vi "pirometer 2.2_MAIN.vi"() -> ()   [LabVIEW 2013]
doc: "Пирометр 2.0, разработан в ЛФВЭ ОИЯИ 2013"
uses:
  pirometer typedef1.ctl
  <vilib>/Utility/error.llb/DialogType.ctl
  <vilib>/Instr/_visa.llb/VISA Configure Serial Port (Instr).vi
  <vilib>/ptbypt/NI_PtbyPt.lvlib
panel:
  in  "Бод.":u32=9600
  out "Ошибка  прибора":bool
  in  "Недопустимая \nразница между\n показаниями":u8=100
  in  "Снимок экрана":bool
  in  "Мин\n  d/dt":dbl=-0.02 min=-200.0 max=200.0 step=0.01 format="%#.3g"
  in  "Макс\n  d/dt":dbl=0.02 min=-200.0 max=200.0 step=0.01 format="%#.3g"
  out "d/dt right scale":dbl(slide) min=-0.20900000000000002 max=0.196 scale=-0.02..0.02
  out "gradusnik 2":dbl(slide) scale=10.0..35.0
  in  "Мин. Т":i8=10
  in  "Stop":bool
  out "gradusnik":dbl(slide) scale=10.0..35.0
  in  "Усреднение d/dt":u16=25
  in  "Усреднение T по":u8=50
  out "Средняя T":dbl format="%0.2f"
  out "d/dt":dynamicdata(graph)
  in  "Макс.Т":i8=35
  out "Температура":dynamicdata(graph)
  in  "Запись в файл":bool
  out "сек.":string="20"
  out "мин.":string="3"
  out "часы":string
  in  "xScale +":bool
  in  "Добавить время":dbl(ring)=60.0 items=["1 сек."=1.0, "10 сек."=10.0, "1 мин."=60.0, "5 мин."=300.0, "10 мин."=600.0]
  in  "xScale -":bool
  out "Текущая T":dbl format="%0.2f"
  in  "Порт":refnum<visa-resource-name>="COM4"
  out "Соединение":bool
  out "Чтение":bool
  out "Расположение файла":path=path "Запись в файл не включена..."
  out "d/dt":dbl format="%#.3f"
  in  "2 или 1 ?":bool=TRUE
  out "Exitting":string="Остановка программы..."
  in  "index of current arr element":i32
  out "i":i32
  in  "number of data sample":u64
  out "refnum out":refnum<file>
  in  "fl_1":bool
  out "Temper.":dbl
  out "Err msg":string=" INSTRUCTIONS:\r\rNormal Use:  When using subVIs that incorporate the error in/error out (or error I/O) structure, place this handler where you want to inform the user of an error, typically at the end of the I/O data path, as the last action of the program.  If the error in error? is ERROR, the handler creates a message describing the error and its source.  If the type of dialog = 1 (default), the message is displayed to the user, who can only acknowedge it.  If the type = 2, the user can acknowledge the message or abort execution; aborting a program with active I/O is not recommended.  If the type = 0, no message is displayed; this is used to process the error programmatically, and the error out cluster elements are wired to individual terminals for that reason.  \r\rOther Use:\n\r\nlocal testing.  To test the error code of a subVI or function that does not have the error I/O structure, you can wire its error code and a source string to the local error code and error source inputs.  If error in error? indicates no error and error code is not equal to 0, the local code and source are substituted for the error in values, and error? is set TRUE (ERROR)."
  # "Показывать два графика?"
  # "°С"
  # "°С"
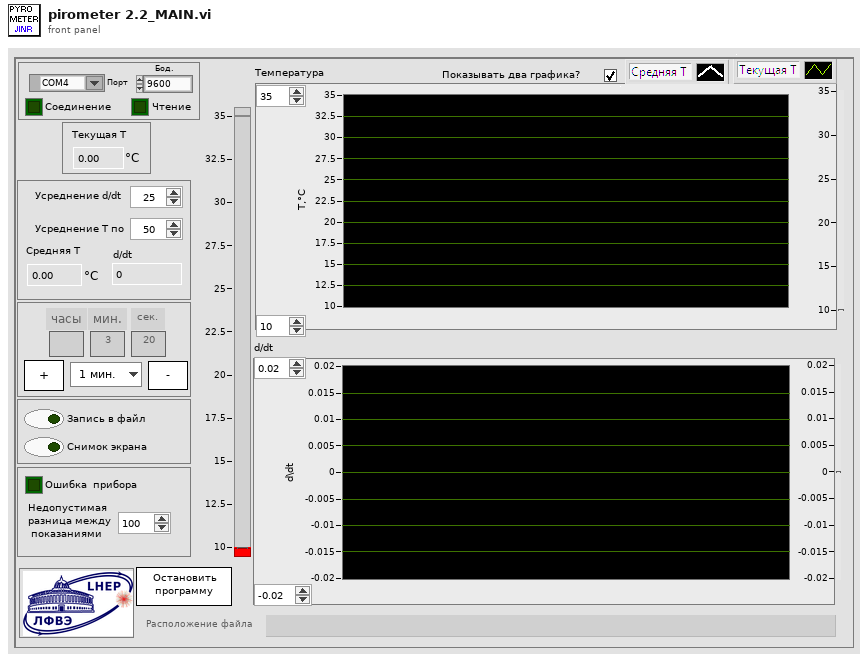
[diagram p1: front panel]
types:
  T1 = typedef "pirometer typedef1.ctl" = enum16{"Initialize", "Read port", "Averaging", "Create graph", "Save to file", "Stop", "ScreenCapture", "Err handle"}
  T2 = typedef "DialogType.ctl" = u16
  T3 = typedef "imagedata.ctl" = cluster{"image type":i32, "image depth":i32, "image":u8[], "mask":u8[], "colors":u32[], "Rectangle":cluster{"left":i16, "top":i16, "right":i16, "bottom":i16}}
  T4 = typedef "LVDateTimeRec.ctl" = cluster{"fractional second":dbl, "second":i32, "minute":i32, "hour":i32, "day of month":i32, "month":i32, "year":i32, "day of week":i32, "day of year":i32, "DST":i32}
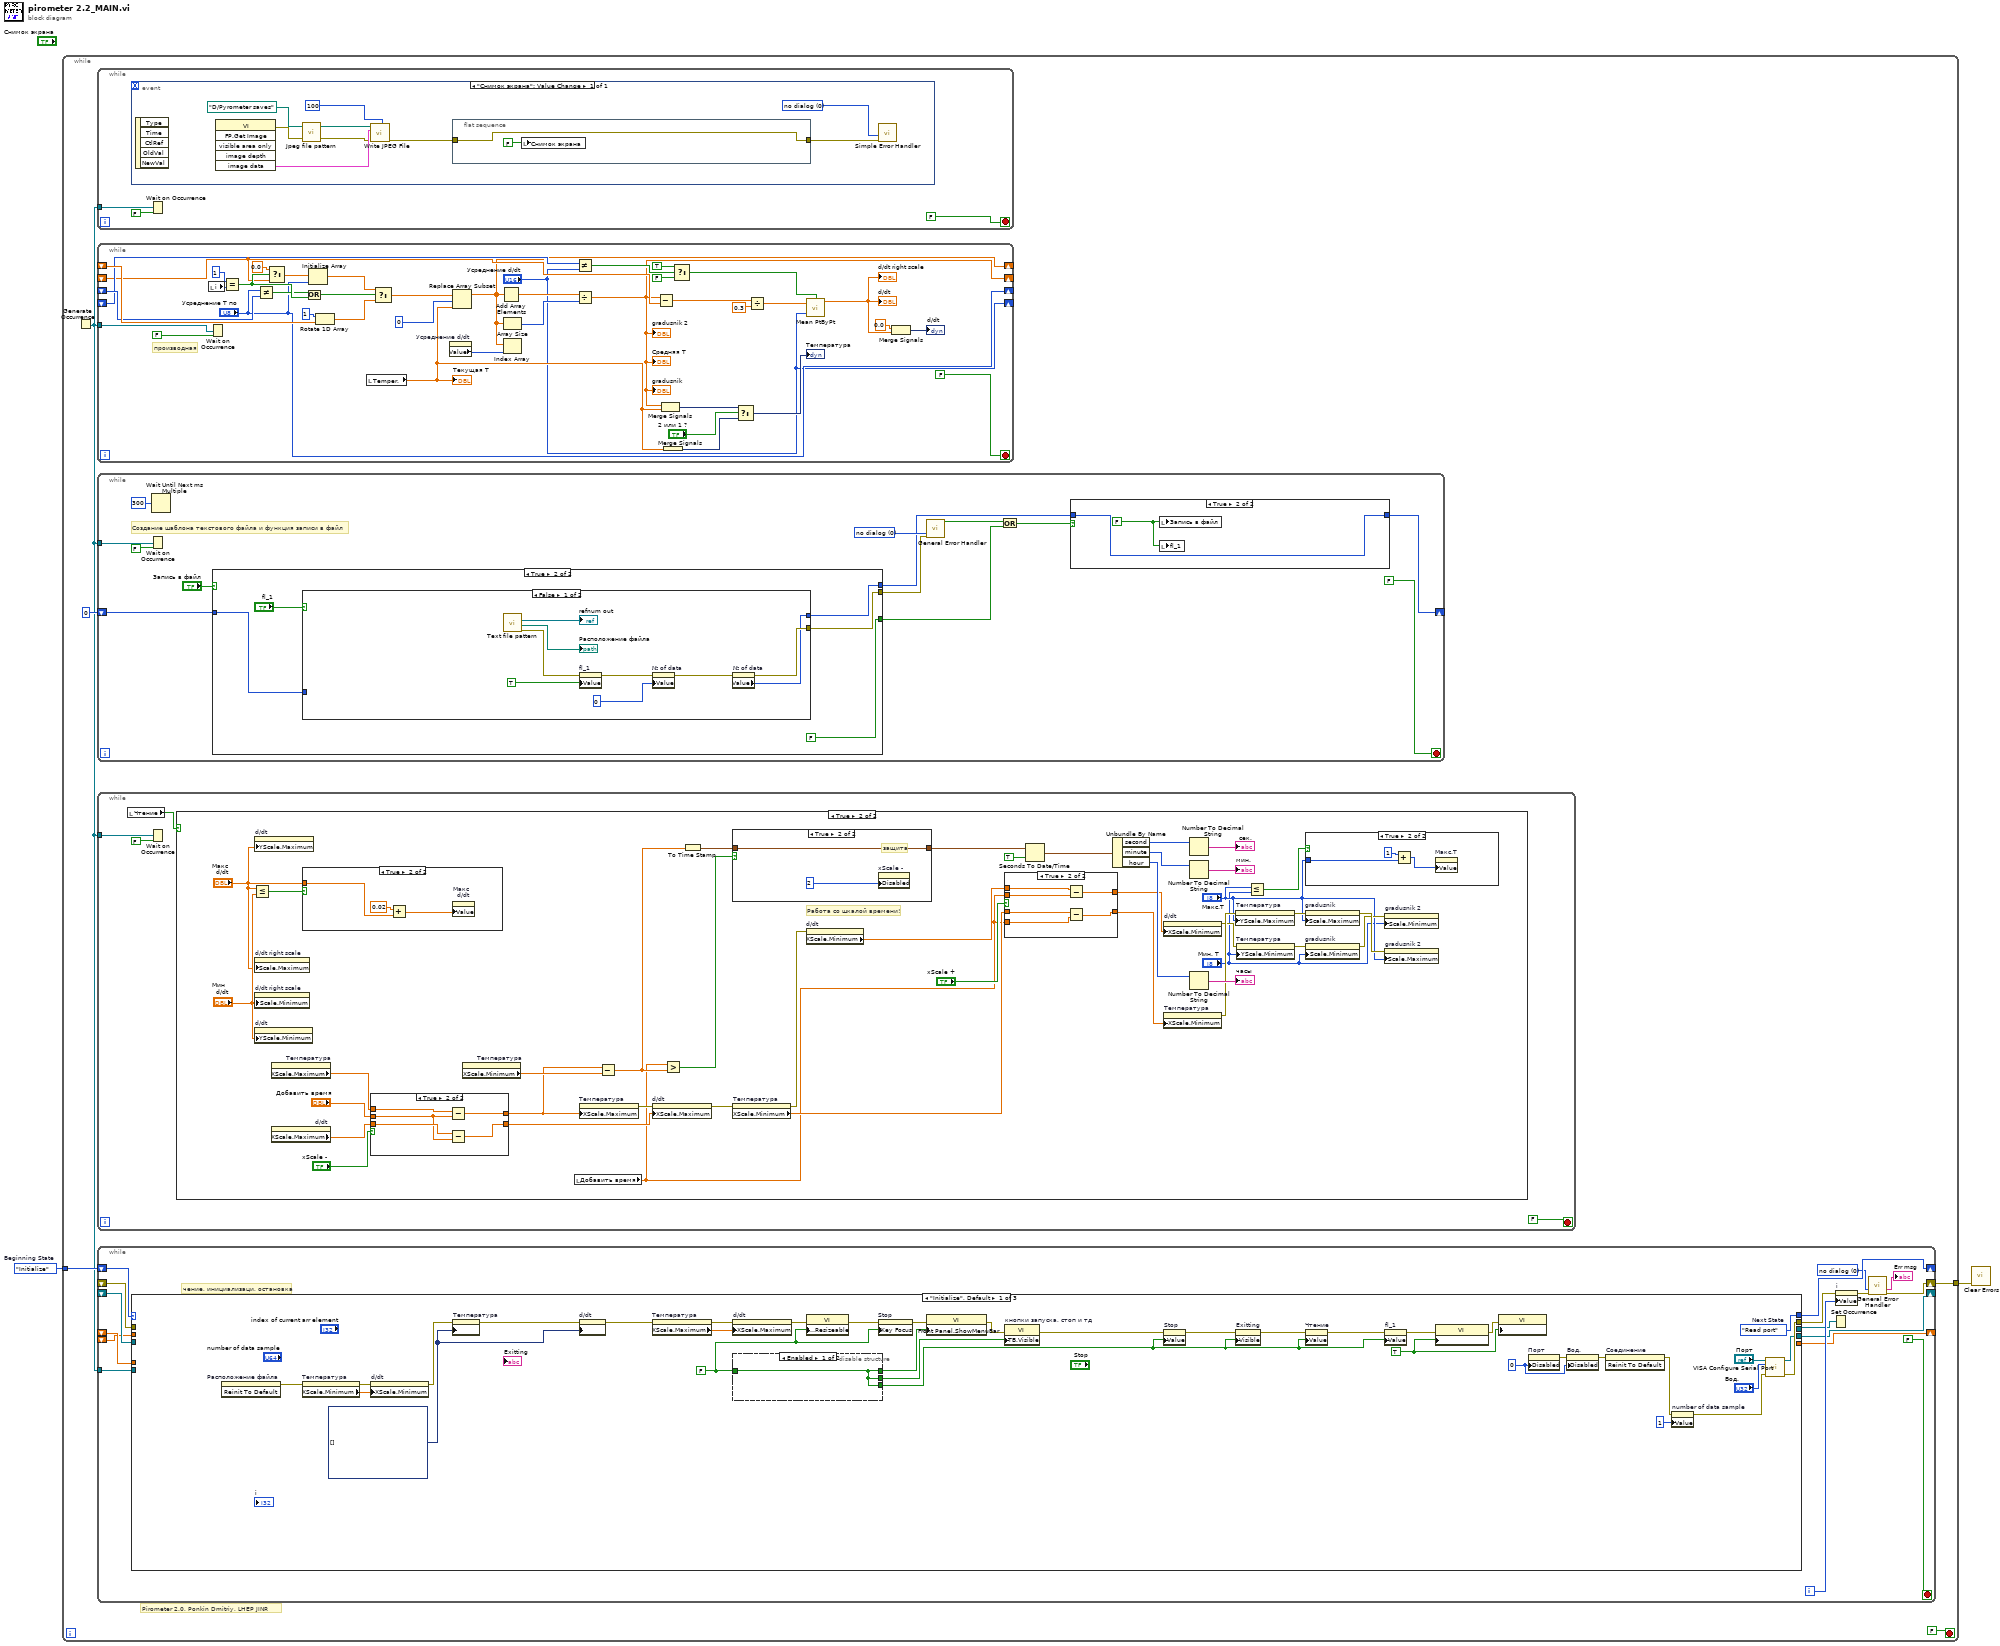
[diagram p0: block diagram]
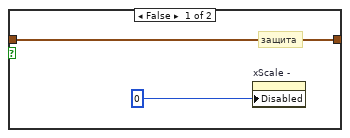
[diagram p5: hidden frame]
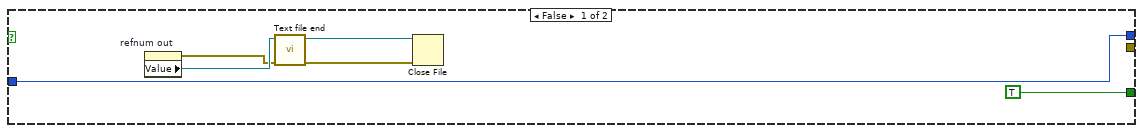
[diagram p9: hidden frame]
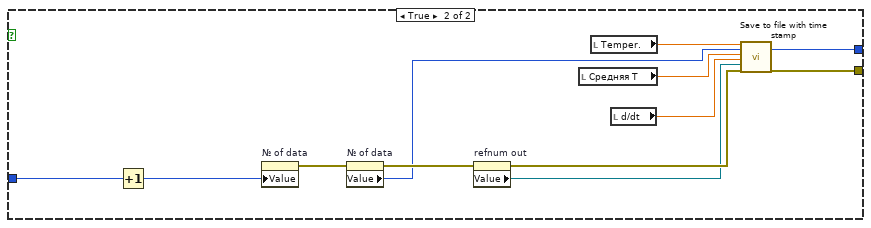
[diagram p10: hidden frame]
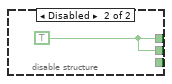
[diagram p11: hidden frame]
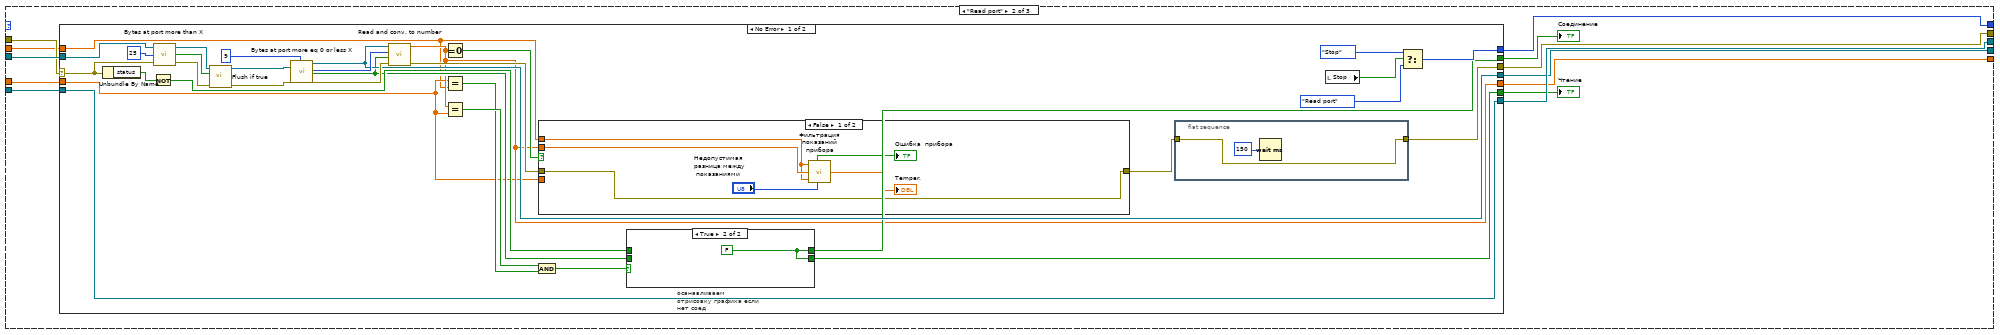
[diagram p12: hidden frame]
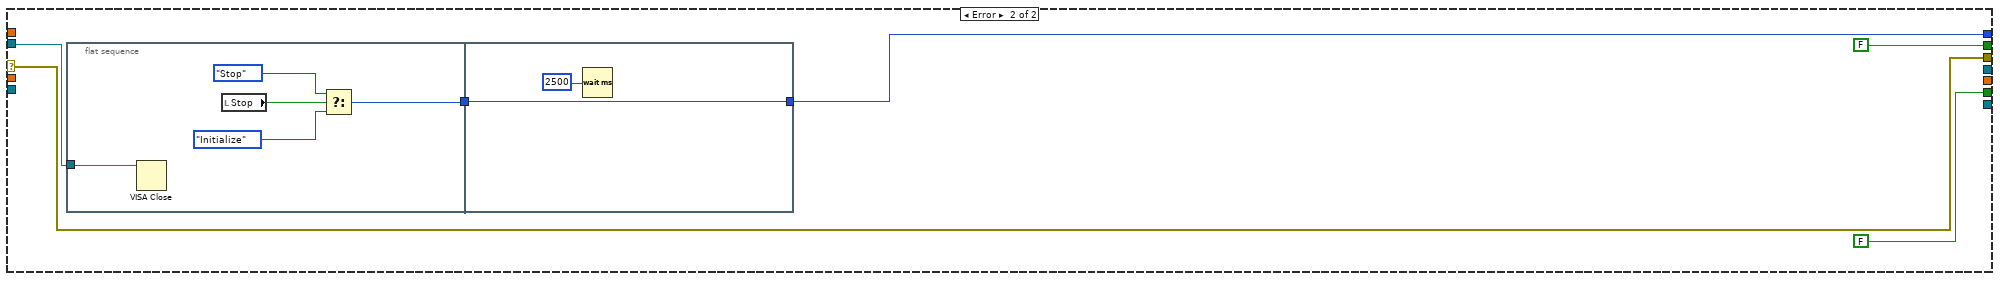
[diagram p15: hidden frame]
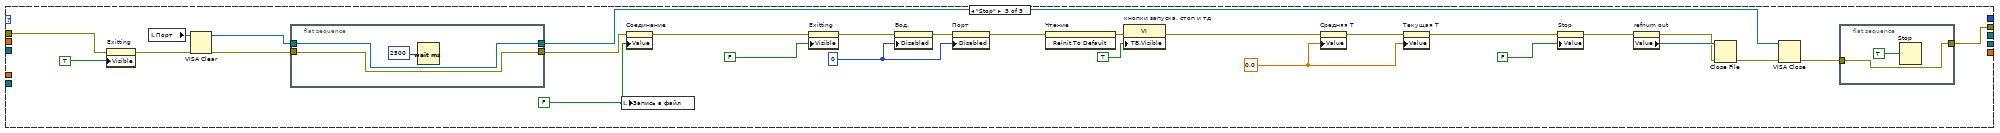
[diagram p16: hidden frame]
diagram:
  w2 = pirometer_typedef1."Initialize"  # Beginning State
  n1 = while {
    tunnel: w2 -> [w7]
    tunnel: [w5] -> w1
    stop <- FALSE stop-if-true
    # "Pirometer 2.0, Ponkin Dmitriy, LHEP JINR"
    n2 = Generate Occurrence() -> (w3:refnum<k4>)
    n3 = while {
      tunnel: w3 -> [w8]
      stop <- FALSE stop-if-true
      n4 = event shown="[0] \"Снимок экрана\": Value Change" {
        selector: _ -> [_]
        dyn-events: _ -> [_]
        timeout: _ -> [_]
        event "Снимок экрана": Value Change {
          w12 = T2 0 items=["no dialog", "OK message", "continue or stop message", "OK message + warnings", "continue/stop + warnings"] ("type of dialog (OK msg:1)")
          n5 = event-data() -> ()  [unwired: 6 out]
          n6 = invoke class="VI" method="FP.Get Image"() -> (error out=w17:errorcluster, "image data"=w18:T3)  [unwired: 6 in, 4 out]
          n7 = call "Jpeg file pattern.vi"("path"=path "D:/Pyrometer saves", "error in"=w17) -> ("path to JPG file"=w16:path, "error out"=w15:errorcluster)  [unwired: 6 out]
          n8 = call <vilib>:"Write JPEG File.vi"("quality (80)"=100, "error in (no error)"=w15, "image data"=w18, "path to JPEG file"=w16) -> ("error out"=w13:errorcluster)  [unwired: 7 out]
          n9 = flat-sequence {
            tunnel: w13 -> [w20]
            tunnel: [w20] -> w11
            frame #0 {
              n10 = local write "Снимок экрана"(FALSE ("Снимок экрана")) -> ()
            }
          }
          n11 = call <vilib>:"Simple Error Handler.vi"("type of dialog (OK msg:1)"=w12, "error in (no error)"=w11) -> ()  [unwired: 8 out]
        }
      }
      n12 = Wait on Occurrence(1:FALSE ("ignore previous (T)"), 2:w8) -> ()  [unwired: 1 in, 1 out]
    }
    n13 = while {
      shift-right: [w24] -> _
      shift-left: _ -> [w62]
      tunnel: w3 -> [w59]
      shift-right: ["Усреднение T по"] -> _
      shift-left: _ -> [w54]
      shift-right: [w30] -> _
      shift-left: _ -> [w31]
      shift-right: ["Усреднение d/dt"] -> _
      shift-left: _ -> [w33]
      stop <- FALSE stop-if-true
      # "производная"
      n14 = local read "i"() -> (w27:i32)
      n15 = Wait on Occurrence(1:FALSE ("ignore previous (T)"), 2:w59) -> ()  [unwired: 1 in, 1 out]
      n16 = Equal?(x=1 ("y"), y=w27) -> (x = y?=w52:bool)
      n17 = Not Equal?(x="Усреднение T по", y=w54) -> (x != y?=w49:bool)
      n18 = Select(t=0.0, s=w52, f=w31) -> (s? t:f=w50:dbl)
      n19 = Or(x=w49, y=w52) -> (x .or. y?=w48:bool)
      n20 = Initialize Array(w50, "Усреднение T по") -> (w43:dbl[])
      n21 = Rotate 1D Array(1:w62, 2:1 ("n")) -> (0:w45:dbl[])
      n22 = local read "Temper."() -> (w40:dbl)
      "Текущая T" <- w40
      n23 = Select(t=w43, s=w48, f=w45) -> (s? t:f=w26:dbl[])
      n24 = property on="Усреднение d/dt" class="DigNum (strict)"() -> ("Value"=w25:u16)  [unwired: 2 in, 2 out]
      n25 = Replace Array Subset(array=w26, new element=w40, index=0) -> (w24:dbl[])
      n26 = Add Array Elements(numeric array=w24) -> (sum=w53:dbl)
      n27 = Array Size(array=w24) -> (size(s)=w29:i32)
      n28 = Index Array(array=w24, index=w25) -> ()  [unwired: 1 out]
      n29 = Not Equal?(x=w33, y="Усреднение d/dt") -> (x != y?=w34:bool)
      n30 = Divide(x=w53, y=w29) -> (x/y=w30:dbl)
      "Средняя T" <- w30
      "gradusnik" <- w30
      "gradusnik 2" <- w30
      n31 = Subtract(x=w30, y=w31) -> (x-y=w42:dbl)
      n32 = Merge Signals(w30, w40) -> (w58:dynamicdata)
      n33 = Merge Signals(w40) -> (w57:dynamicdata)
      n34 = Select(t=TRUE ("initialize"), s=w34, f=FALSE ("initialize")) -> (s? t:f=w32:bool)
      n35 = Select(t=w58, s="2 или 1 ?", f=w57) -> (s? t:f=→"Температура":dynamicdata)
      n36 = Divide(x=w42, y=0.3 ("dT")) -> (x/y=w37:dbl)
      n37 = call <vilib>:"Mean PtByPt.vi"("x"=w37, "sample length"="Усреднение d/dt", "initialize"=w32) -> ("mean"=w38:dbl)  [unwired: 2 out]
      "d/dt" <- w38
      "d/dt right scale" <- w38
      n38 = Merge Signals(0.0 ("f"), w38) -> (→"d/dt":dynamicdata)
    }
    n39 = while {
      shift-right: [w136] -> _
      shift-left: u64 0 ("number of data sample out") -> [w144]
      tunnel: w3 -> [w143]
      stop <- FALSE stop-if-true
      w140 = T2 0 items=["no dialog", "OK message", "continue or stop message", "OK message + warnings", "continue/stop + warnings"] ("type of dialog (OK msg:1)")
      # "Создание шаблона текстового файла и функция записи в файл"
      n40 = Wait on Occurrence(1:FALSE ("ignore previous (T)"), 2:w143) -> ()  [unwired: 2 out]
      n41 = Wait Until Next ms Multiple(millisecond multiple=u32 300 ("milliseconds to wait")) -> ()  [unwired: 1 out]
      n42 = case shown="True" "Запись в файл" {
        tunnel: [_ w158] -> w138
        tunnel: [w153 w156] -> w137
        tunnel: w144 -> [w153 w155]
        tunnel: [TRUE ("save to file ?") FALSE ("save to file ?")] -> w133
        frame False {
          n43 = property on="refnum out" class="Ref (strict)"() -> (error out=w150:errorcluster, "Value"=w151:refnum<file>)  [unwired: 2 in, 1 out]
          n44 = call "Text file end.vi"("error in"=w150, "refnum file"=w151) -> ("error out"=w152:errorcluster, "refnum out"=w149:refnum<file>)  [unwired: 1 in, 7 out]
          n45 = Close File(refnum=w149, error in=w152) -> ()  [unwired: 2 out]
        }
        frame True {
          n46 = case shown="False" "fl_1" {
            tunnel: [w160 w175] -> w158
            tunnel: [w159 w171] -> w156
            tunnel: w155 -> [_ w178]
            frame False {
              n47 = call "Text file pattern.vi"() -> ("error out"=w166:errorcluster, "selected path"=→"Расположение файла":path, "refnum out"=→"refnum out":refnum<file>)  [unwired: 4 in, 5 out]
              n48 = property on="fl_1" class="Bool (strict)"(error in=w166, "Value"=TRUE ("fl_1")) -> (error out=w163:errorcluster)  [unwired: 1 in, 1 out]
              n49 = property on="№ of data" class="DigNum (strict)"(error in=w163, "Value"=u64 0 ("number of data sample")) -> (error out=w161:errorcluster)  [unwired: 1 in, 1 out]
              n50 = property on="№ of data" class="DigNum (strict)"(error in=w161) -> (error out=w160:errorcluster, "Value"=w159:u64)  [unwired: 1 in, 1 out]
            }
            frame True {
              n51 = Increment(x=w178) -> (x+1=w179:u64)
              n52 = property on="№ of data" class="DigNum (strict)"("Value"=w179) -> (error out=w176:errorcluster)  [unwired: 2 in, 1 out]
              n53 = property on="№ of data" class="DigNum (strict)"(error in=w176) -> (error out=w177:errorcluster, "Value"=w172:u64)  [unwired: 1 in, 1 out]
              n54 = property on="refnum out" class="Ref (strict)"(error in=w177) -> (error out=w174:errorcluster, "Value"=w173:refnum<file>)  [unwired: 1 in, 1 out]
              n55 = local read "Средняя T"() -> (w169:dbl)
              n56 = local read "Temper."() -> (w170:dbl)
              n57 = local read "d/dt"() -> (w168:dbl)
              n58 = call "Save to file with time stamp.vi"("T in"=w170, "number of data sample"=w172, "Average in"=w169, "d/dt in"=w168, "refnum file"=w173, "error in"=w174) -> ("number of data sample out"=w171:u64, "error out"=w175:errorcluster)  [unwired: 12 out]
            }
          }
        }
      }
      n59 = call <vilib>:"General Error Handler.vi"("type of dialog (OK msg:1)"=w140, "error in (no error)"=w138) -> ("error?"=w135:bool)  [unwired: 13 out]
      n60 = Or(x=w135, y=w133) -> (x .or. y?=w134:bool)
      n61 = case shown="True" w134 {
        tunnel: w137 -> [w145 w146]
        tunnel: [w145 w146] -> w136
        frame False {
        }
        frame True {
          w147 = FALSE ("save to file ?")
          n62 = local write "Запись в файл"(w147) -> ()
          n63 = local write "fl_1"(w147) -> ()
        }
      }
    }
    n64 = while {
      tunnel: w3 -> [w63]
      stop <- FALSE stop-if-true
      n65 = local read "Чтение"() -> (w65:bool)
      n66 = Wait on Occurrence(1:FALSE ("ignore previous (T)"), 2:w63) -> ()  [unwired: 1 in, 1 out]
      n67 = case shown="True" w65 {
        frame False {
        }
        frame True {
          # "Работа со шкалой времени!"
          n68 = Less Or Equal?(x="Макс\n  d/dt", y="Мин\n  d/dt") -> (x <= y?=w75:bool)
          n69 = property on="d/dt" class="WFChart (strict)"("YScale.Maximum"="Макс\n  d/dt") -> ()  [unwired: 2 in, 2 out]
          n70 = property on="d/dt right scale" class="Slide (strict)"("Scale.Maximum"="Макс\n  d/dt") -> ()  [unwired: 2 in, 2 out]
          n71 = property on="d/dt right scale" class="Slide (strict)"("Scale.Minimum"="Мин\n  d/dt") -> ()  [unwired: 2 in, 2 out]
          n72 = property on="d/dt" class="WFChart (strict)"("YScale.Minimum"="Мин\n  d/dt") -> ()  [unwired: 2 in, 2 out]
          n73 = property on="Температура" class="WFChart (strict)"() -> ("XScale.Maximum"=w95:dbl)  [unwired: 2 in, 2 out]
          n74 = property on="d/dt" class="WFChart (strict)"() -> ("XScale.Maximum"=w87:dbl)  [unwired: 2 in, 2 out]
          n75 = case shown="True" w75 {
            tunnel: "Макс\n  d/dt" -> [_ w112]
            frame False {
            }
            frame True {
              n76 = Add(x=0.02, y=w112) -> (x+y=w110:dbl)
              n77 = property on="Макс\n  d/dt" class="DigNum (strict)"("Value"=w110) -> ()  [unwired: 2 in, 2 out]
            }
          }
          n78 = case shown="True" "xScale -" {
            tunnel: w95 -> [w118 w122]
            tunnel: [w118 w123] -> w88
            tunnel: "Добавить время" -> [_ w120]
            tunnel: w87 -> [w117 w121]
            tunnel: [w117 w119] -> w86
            frame False {
            }
            frame True {
              n79 = Subtract(x=w122, y=w120) -> (x-y=w123:dbl)
              n80 = Subtract(x=w121, y=w120) -> (x-y=w119:dbl)
            }
          }
          n81 = property on="Температура" class="WFChart (strict)"() -> ("XScale.Minimum"=w93:dbl)  [unwired: 2 in, 2 out]
          n82 = local read "Добавить время"() -> (w67:dbl)
          n83 = property on="Температура" class="WFChart (strict)"("XScale.Maximum"=w88) -> (error out=w83:errorcluster)  [unwired: 2 in, 1 out]
          n84 = Subtract(x=w88, y=w93) -> (x-y=w98:dbl)
          n85 = property on="d/dt" class="WFChart (strict)"(error in=w83, "XScale.Maximum"=w86) -> (error out=w82:errorcluster)  [unwired: 1 in, 1 out]
          n86 = Greater?(x=w67, y=w98) -> (0:w97:bool)
          n87 = To Time Stamp(1:w98) -> (0:w91:timestamp)
          n88 = case shown="True" w97 {
            tunnel: [w113 w115] -> w90
            tunnel: w91 -> [w113 w115]
            frame False {
              # "защита"
              n89 = property on="xScale -" class="Bool"("Disabled"=u8 0) -> ()  [unwired: 2 in, 2 out]
            }
            frame True {
              # "защита"
              n90 = property on="xScale -" class="Bool"("Disabled"=u8 2) -> ()  [unwired: 2 in, 2 out]
            }
          }
          n91 = property on="Температура" class="WFChart (strict)"(error in=w82) -> (error out=w80:errorcluster, "XScale.Minimum"=w81:dbl)  [unwired: 1 in, 1 out]
          n92 = property on="d/dt" class="WFChart (strict)"(error in=w80) -> ("XScale.Minimum"=w85:dbl)  [unwired: 1 in, 2 out]
          n93 = case shown="True" "xScale +" {
            tunnel: w81 -> [w125 w131]
            tunnel: [w125 w130] -> w89
            tunnel: w67 -> [_ w129]
            tunnel: w85 -> [w124 w128]
            tunnel: w67 -> [_ w127]
            tunnel: [w124 w126] -> w84
            frame False {
            }
            frame True {
              n94 = Subtract(x=w128, y=w127) -> (x-y=w126:dbl)
              n95 = Subtract(x=w131, y=w129) -> (x-y=w130:dbl)
            }
          }
          n96 = Seconds To Date/Time(time stamp (now)=w90, to UTC (F)=TRUE) -> (date time rec=w100:T4)
          n97 = Unbundle By Name(w100) -> ("second"=w101:i32, "minute"=w102:i32, "hour"=w103:i32)
          n98 = property on="d/dt" class="WFChart (strict)"("XScale.Minimum"=w84) -> (error out=w78:errorcluster)  [unwired: 2 in, 1 out]
          n99 = property on="Температура" class="WFChart (strict)"("XScale.Minimum"=w89) -> (error out=w79:errorcluster)  [unwired: 2 in, 1 out]
          n100 = Number To Decimal String(number=w101) -> (decimal integer string=→"сек.":string)  [unwired: 1 out]
          n101 = Number To Decimal String(number=w102) -> (decimal integer string=→"мин.":string)  [unwired: 1 out]
          n102 = Number To Decimal String(number=w103) -> (decimal integer string=→"часы":string)  [unwired: 1 out]
          n103 = property on="Температура" class="WFChart (strict)"(error in=w79, "YScale.Maximum"="Макс.Т") -> (error out=w77:errorcluster)  [unwired: 1 in, 1 out]
          n104 = property on="Температура" class="WFChart (strict)"(error in=w78, "YScale.Minimum"="Мин. Т") -> (error out=w76:errorcluster)  [unwired: 1 in, 1 out]
          n105 = Less Or Equal?(x="Макс.Т", y="Мин. Т") -> (x <= y?=w70:bool)
          n106 = case shown="True" w70 {
            tunnel: "Макс.Т" -> [_ w109]
            frame False {
            }
            frame True {
              n107 = Add(x=i8 1, y=w109) -> (x+y=w107:i8)
              n108 = property on="Макс.Т" class="DigNum (strict)"("Value"=w107) -> ()  [unwired: 2 in, 2 out]
            }
          }
          n109 = property on="gradusnik" class="Slide (strict)"(error in=w77, "Scale.Maximum"="Макс.Т") -> (error out=w74:errorcluster)  [unwired: 1 in, 1 out]
          n110 = property on="gradusnik" class="Slide (strict)"(error in=w76, "Scale.Minimum"="Мин. Т") -> (error out=w73:errorcluster)  [unwired: 1 in, 1 out]
          n111 = property on="gradusnik 2" class="Slide (strict)"(error in=w73, "Scale.Minimum"="Мин. Т") -> ()  [unwired: 1 in, 2 out]
          n112 = property on="gradusnik 2" class="Slide (strict)"(error in=w74, "Scale.Maximum"="Макс.Т") -> ()  [unwired: 1 in, 2 out]
        }
      }
    }
    n113 = while {
      shift-right: [w195] -> _
      shift-left: w7 -> [w196]
      shift-right: [w193] -> w5
      shift-left: _ -> [w190]
      tunnel: w3 -> [w186]
      shift-right: [w184] -> _
      shift-left: _ -> [w183]
      shift-right: [w182] -> _
      shift-left: _ -> [w181]
      shift-left: _ -> [w180]
      i -> [w189]
      stop <- FALSE stop-if-true
      w192 = T2 0 items=["no dialog", "OK message", "continue or stop message", "OK message + warnings", "continue/stop + warnings"] ("type of dialog (OK msg:1)")
      # "чение, инициализаци, остановка"
      n114 = case shown="\"Initialize\", Default" w196 {
        tunnel: [w225 w245 _] -> w195
        tunnel: [w224 w240 w308] -> w188
        tunnel: w190 -> [_ w237 w330]
        tunnel: w186 -> [_ w242 _]
        tunnel: [_ w243 _] -> w185
        tunnel: [w222 w238 _] -> w184
        tunnel: w183 -> [_ w239 _]
        tunnel: [_ w236 _] -> w182
        tunnel: w181 -> [_ w235 _]
        tunnel: w180 -> [_ w234 _]
        frame "Initialize", Default {
          w223 = dynamicdata[] [] ("History Data")
          w225 = pirometer_typedef1."Read port"  # Next State
          w216 = TRUE ("Front Panel Window:Minimizable")
          w204 = FALSE ("Front Panel Window:Resizable")
          w213 = u8 0 ("Disabled")
          n115 = invoke on="Расположение файла" class="Path" method="Reinit To Default"() -> (error out=w205:errorcluster)  [unwired: 3 in, 2 out]
          n116 = property on="Температура" class="WFChart (strict)"(error in=w205) -> (error out=w206:errorcluster, "XScale.Minimum"=w211:dbl)  [unwired: 1 in, 1 out]
          n117 = property on="d/dt" class="WFChart (strict)"(error in=w206, "XScale.Minimum"=w211) -> (error out=w207:errorcluster)  [unwired: 1 in, 1 out]
          n118 = property on="Температура" class="WFChart (strict)"(error in=w207, "History Data"=w223) -> (error out=w209:errorcluster)  [unwired: 1 in, 1 out]
          n119 = property on="d/dt" class="WFChart (strict)"(error in=w209, "History Data"=w223) -> (error out=w208:errorcluster)  [unwired: 1 in, 1 out]
          n120 = property on="Температура" class="WFChart (strict)"(error in=w208) -> (error out=w197:errorcluster, "XScale.Maximum"=w212:dbl)  [unwired: 1 in, 1 out]
          n121 = property on="d/dt" class="WFChart (strict)"(error in=w197, "XScale.Maximum"=w212) -> (error out=w210:errorcluster)  [unwired: 1 in, 1 out]
          n122 = disable-structure shown="Enabled" {
            disable-tunnel: w204 -> [w232 _]
            disable-tunnel: [w232 _] -> w199
            disable-tunnel: [w232 w233] -> w203
            disable-tunnel: [w232 w233] -> w202
            frame Enabled {
            }
            frame Disabled {
              w233 = TRUE
            }
          }
          n123 = property class="VI"(error in=w210, "Front Panel.Resizeable"=w204) -> (error out=w221:errorcluster)  [unwired: 1 in, 1 out]
          n124 = property on="Stop" class="Bool (strict)"(error in=w221, "Key Focus"=w204) -> (error out=w220:errorcluster)  [unwired: 1 in, 1 out]
          n125 = property class="VI"(error in=w220, "Front Panel.ShowMenuBar"=w203) -> (error out=w219:errorcluster)  [unwired: 1 in, 1 out]
          n126 = property on="кнопки запуска, стоп и тд" class="VI"(error in=w219, "TB.Visible"=w202) -> (error out=w201:errorcluster)  [unwired: 1 in, 1 out]
          n127 = property on="Stop" class="Bool (strict)"(error in=w201, "Value"=w199) -> (error out=w200:errorcluster)  [unwired: 1 in, 1 out]
          n128 = property on="Exitting" class="Str"(error in=w200, "Visible"=w199) -> (error out=w214:errorcluster)  [unwired: 1 in, 1 out]
          n129 = property on="Чтение" class="Bool (strict)"(error in=w214, "Value"=w199) -> (error out=w230:errorcluster)  [unwired: 1 in, 1 out]
          n130 = property on="fl_1" class="Bool (strict)"(error in=w230, "Value"=w199) -> (error out=w218:errorcluster)  [unwired: 1 in, 1 out]
          n131 = property class="VI"(error in=w218, "Front Panel.Minimizeable"=w216) -> (error out=w215:errorcluster)  [unwired: 1 in, 1 out]
          n132 = property class="VI"(error in=w215, "Front Panel.TitleBarVis"=w216) -> ()  [unwired: 1 in, 2 out]
          n133 = property on="Порт" class="VISAName"("Disabled"=w213) -> (error out=w198:errorcluster)  [unwired: 2 in, 1 out]
          n134 = property on="Бод." class="DigNum (strict)"(error in=w198, "Disabled"=w213) -> (error out=w226:errorcluster)  [unwired: 1 in, 1 out]
          n135 = invoke on="Соединение" class="Bool (strict)" method="Reinit To Default"(error in=w226) -> (error out=w229:errorcluster)  [unwired: 2 in, 2 out]
          n136 = property on="number of data sample" class="DigNum (strict)"(error in=w229, "Value"=u64 1 ("number of data sample")) -> (error out=w217:errorcluster)  [unwired: 1 in, 1 out]
          n137 = call-poly "VISA Configure Serial Port"("VISA resource name"="Порт", "baud rate (9600)"="Бод.", "error in (no error)"=w217) -> ("VISA resource name out"=w222:refnum<visa-resource-name>, "error out"=w224:errorcluster)  [unwired: 3 in, 8 out]
        }
        frame "Read port" {
          n138 = case shown="No Error" w237 {
            selector: w237 -> [w261 w295]
            tunnel: [w258 w295] -> w240
            tunnel: [w274 w293] -> w245
            tunnel: [w254 FALSE] -> w244
            tunnel: [w252 FALSE ("Reading data")] -> w241
            tunnel: [w265 _] -> w243
            tunnel: w242 -> [w265 _]
            tunnel: w239 -> [w257 w290]
            tunnel: [w256 _] -> w238
            tunnel: [w248 _] -> w236
            tunnel: w235 -> [w247 _]
            tunnel: w234 -> [w246 _]
            frame No Error {
              n139 = Unbundle By Name(w261) -> ("status"=w260:bool)
              n140 = Not(x=w260) -> (.not. x?=w255:bool)
              n141 = call "Bytes at port more than X.vi"("error IO"=w261, "X"=u32 25, "port in"=w257) -> ("error out"=w273:errorcluster, "Bytes at port > X"=w272:bool, "port out"=w271:refnum<visa-resource-name>)
              n142 = call "Flush if true.vi"("error in"=w273, "Bytes at port > X"=w272, "port in"=w271) -> ("error out"=w270:errorcluster, "port out"=w269:refnum<visa-resource-name>)  [unwired: 7 out]
              n143 = call "Bytes at port more eq 0 or less X.vi"("serial ref  name"=w269, "error IO"=w270, "X"=u32 9) -> ("serial out"=w256:refnum<visa-resource-name>, "Num. of Bytes at Port"=w266:u32, "Bytes at port <X or = 0?"=w253:bool, "error out"=w267:errorcluster)  [unwired: 1 in, 12 out]
              n144 = call "Read and conv. to number.vi"("error in"=w267, "Bytes at port <X or = 0?"=w253, "Num. of Bytes at Port"=w266, "port"=w256) -> ("error out"=w263:errorcluster, "Temper."=w248:dbl)  [unwired: 6 out]
              n145 = Equal To 0?(x=w248) -> (x = 0?=w264:bool)
              n146 = Equal?(x=w247, y=w246) -> (x = y?=w249:bool)
              n147 = Equal?(x=w248, y=w247) -> (x = y?=w250:bool)
              n148 = And(x=w250, y=w249) -> (x .and. y?=w251:bool)
              n149 = case shown="False" w264 {
                tunnel: w263 -> [w288 w289]
                tunnel: [w288 w289] -> w259
                tunnel: w248 -> [w284 _]
                tunnel: w247 -> [_ _]
                tunnel: w246 -> [w283 _]
                frame False {
                  n150 = call "Фильтрация показаний прибора.vi"("Предпредыдущее показание"=w283, "Текущее показание"=w284, "Предыдущее показание"=w283, "Разница между \nпоказаниями прибора"="Недопустимая \nразница между\n показаниями") -> ("Ошибка \nприбора"=→"Ошибка  прибора":bool, "Отфильтрован.\nвеличина"=→"Temper.":dbl)  [unwired: 4 out]
                }
                frame True {
                }
              }
              n151 = case "осанавливаем отрисовку графика если нет соед" shown="True" w251 {
                tunnel: w255 -> [w279 _]
                tunnel: [w279 w280] -> w254
                tunnel: w253 -> [w278 _]
                tunnel: [w278 w280] -> w252
                frame False {
                }
                frame True {
                  w280 = FALSE
                }
              }
              n152 = flat-sequence {
                tunnel: w259 -> [w282]
                tunnel: [w282] -> w258
                frame #0 {
                  n153 = Wait (ms)(milliseconds to wait=u32 150) -> ()  [unwired: 1 out]
                }
              }
              n154 = local read "Stop"() -> (w262:bool)
              n155 = Select(t=pirometer_typedef1."Stop" ("Beginning State"), s=w262, f=pirometer_typedef1."Read port" ("Beginning State")) -> (s? t:f=w274:T1)
            }
            frame Error {
              n156 = flat-sequence {
                tunnel: [w297] -> w294
                tunnel: w290 -> [w296]
                tunnel: [w301] -> w293
                tunnel: w294 -> [w301]
                frame #0 {
                  n157 = VISA Close(VISA resource name=w296) -> ()  [unwired: 1 in, 1 out]
                  n158 = local read "Stop"() -> (w300:bool)
                  n159 = Select(t=pirometer_typedef1."Stop" ("Beginning State"), s=w300, f=pirometer_typedef1."Initialize" ("Beginning State")) -> (s? t:f=w297:T1)
                }
                frame #1 {
                  n160 = Wait (ms)(milliseconds to wait=u32 2500) -> ()  [unwired: 1 out]
                }
              }
            }
          }
          "Соединение" <- w244
          "Чтение" <- w241
        }
        frame "Stop" {
          w314 = 0.0 ("Текущая T")
          w304 = u8 0 ("Disabled")
          w326 = FALSE ("Connected")
          n161 = property on="Exitting" class="Str"(error in=w330, "Visible"=TRUE) -> (error out=w327:errorcluster)  [unwired: 1 in, 1 out]
          n162 = local read "Порт"() -> (w329:refnum<visa-resource-name>)
          n163 = VISA Clear(VISA resource name=w329, error in (no error)=w327) -> (VISA resource name out=w312:refnum<visa-resource-name>, error out=w310:errorcluster)
          n164 = flat-sequence {
            tunnel: w312 -> [w332]
            tunnel: [w332] -> w311
            tunnel: [w331] -> w309
            tunnel: w310 -> [w331]
            frame #0 {
              n165 = Wait (ms)(milliseconds to wait=u32 2500) -> ()  [unwired: 1 out]
            }
          }
          n166 = local write "Запись в файл"(w326) -> ()
          n167 = property on="Соединение" class="Bool (strict)"(error in=w309, "Value"=w326) -> (error out=w305:errorcluster)  [unwired: 1 in, 1 out]
          n168 = property on="Exitting" class="Str"(error in=w305, "Visible"=FALSE) -> (error out=w303:errorcluster)  [unwired: 1 in, 1 out]
          n169 = property on="Бод." class="DigNum (strict)"(error in=w303, "Disabled"=w304) -> (error out=w323:errorcluster)  [unwired: 1 in, 1 out]
          n170 = property on="Порт" class="VISAName"(error in=w323, "Disabled"=w304) -> (error out=w322:errorcluster)  [unwired: 1 in, 1 out]
          n171 = invoke on="Чтение" class="Bool (strict)" method="Reinit To Default"(error in=w322) -> (error out=w324:errorcluster)  [unwired: 2 in, 2 out]
          n172 = property on="кнопки запуска, стоп и тд" class="VI"(error in=w324, "TB.Visible"=TRUE ("Tool Bar:Visible")) -> (error out=w316:errorcluster)  [unwired: 1 in, 1 out]
          n173 = property on="Средняя T" class="DigNum (strict)"(error in=w316, "Value"=w314) -> (error out=w315:errorcluster)  [unwired: 1 in, 1 out]
          n174 = property on="Текущая T" class="DigNum (strict)"(error in=w315, "Value"=w314) -> (error out=w317:errorcluster)  [unwired: 1 in, 1 out]
          n175 = property on="Stop" class="Bool (strict)"(error in=w317, "Value"=FALSE ("Stop")) -> (error out=w319:errorcluster)  [unwired: 1 in, 1 out]
          n176 = property on="refnum out" class="Ref (strict)"(error in=w319) -> (error out=w320:errorcluster, "Value"=w321:refnum<file>)  [unwired: 1 in, 1 out]
          n177 = Close File(refnum=w321, error in=w320) -> (error out=w306:errorcluster)  [unwired: 1 out]
          n178 = VISA Close(VISA resource name=w311, error in (no error)=w306) -> (error out=w307:errorcluster)
          n179 = flat-sequence {
            tunnel: [w335] -> w308
            tunnel: w307 -> [w335]
            frame #0 {
              n180 = Stop(stop? (T)=TRUE) -> ()
            }
          }
        }
      }
      n181 = Set Occurrence(w185) -> ()
      n182 = property on="i" class="DigNum (strict)"(error in=w188, "Value"=w189) -> (error out=w187:errorcluster)  [unwired: 1 in, 1 out]
      n183 = call <vilib>:"General Error Handler.vi"("type of dialog (OK msg:1)"=w192, "error in (no error)"=w187) -> ("message"=→"Err msg":string, "error out"=w193:errorcluster)  [unwired: 12 out]
    }
  }
  n184 = call <vilib>:"Clear Errors.vi"("error in (no error)"=w1) -> ()  [unwired: 7 out]
